vi "New Session SetUp.vi"(8 "error in (no error)":errorcluster, 10 "Stop Refnum":refnum<vi>, 11 "Yokogawa WT1600 in":refnum<class "Yokogawa WT1600.lvclass">) -> (0 "error out":errorcluster, 3 "Yokogawa WT1600 out":refnum<class "Yokogawa WT1600.lvclass">)   [LabVIEW 2014]
uses:
  Yokogawa WT1600.lvclass
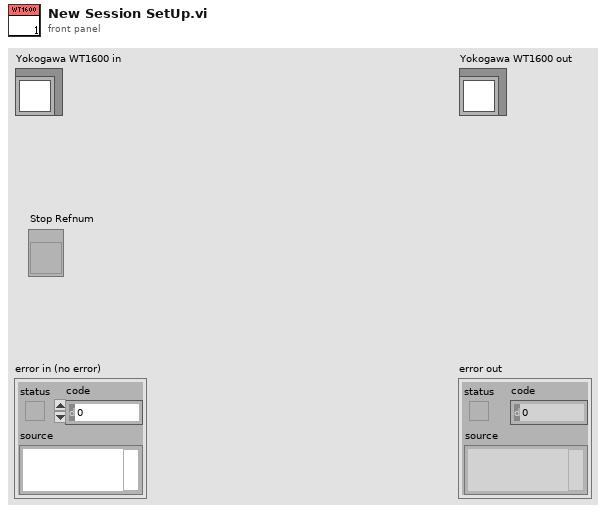
[diagram p1: front panel]
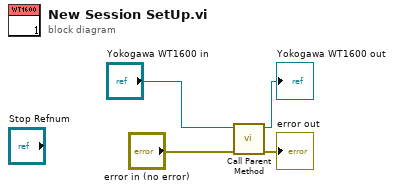
[diagram p0: block diagram]
diagram:
  n1 = call-parent "Call Parent Method"("error in (no error)"="error in (no error)", "Generic Power Analyzer in"="Yokogawa WT1600 in") -> ("error out"=→"error out":errorcluster, "Generic Power Analyzer out"=→"Yokogawa WT1600 out":refnum<class "Yokogawa WT1600.lvclass">)  [unwired: 8 in]
